vi "Front Panel Tyler SYNCHRONIZED.vi"() -> ()   [LabVIEW 2017, in "LD Reading.lvclass"]
uses:
  LD Reading.lvclass
  Experimental Parameters.ctl
  Reference Channel Intensities.ctl
  Sample Channel Intensities.ctl
  Realtime Output.ctl
  Average Data.ctl
  LD Reading.lvclass/LD Reading.ctl
  MCTypedef.ctl
  <vilib>/Instr/_visa.llb/VISA Configure Serial Port (Instr).vi
  <vilib>/Utility/file.llb/Write Delimited Spreadsheet (string).vi
  <vilib>/Utility/inputDevices.llb/keyboardAcquire.vi
panel:
  in  "Experimental Controls":enum32{"Page 1", "Page 2"}(tab)
  in  "Collect Data":bool
  out "Running":bool
  in  "Save Measurements?":bool
  in  "Stop and Discard \nMeasurement":bool
  in  "Output Filename (stem)":path
  out "Finished":bool
  in  "Selected Reference Channel":enum32{"Channel 1", "Channel 2", "Channel 3"}(radio)
  in  "Selected Sample Channel":enum32{"Channel 1", "Channel 2", "Channel 3"}(radio)
  in  "Data Collection Mode":enum32{"Reference", "Sample"}(radio)
  in  "Export Data":bool
  in  "Enable Translation Stage":bool
  in  "Shutter Control":bool
  out "error out":errorcluster
  in  "clear":bool
  in  "sp33d":dbl(knob)=0.5 step=0.5 scale=0.5..1.0
  out "read buffer":string
  out "Data Collection Progress":u8(slide) scale=0.0..100.0
  out "Current Phase":string
  in  "?":T1(tab)
  out "Diode/PMT":cluster{dbl[], dbl[]}(graph)
  out "RMS Voltage":cluster{dbl[], dbl[]}(graph)
  out "Photodiode Voltage  (V)":cluster{dbl[], dbl[]}(graph)
  out "PMT Voltage":cluster{dbl[], dbl[]}(graph)
  out "Reference Averages":T2
  out "Sample Averages":T2
  out "Realtime Output":T3
  out "Sample Analysis":T4
  out "Reference Analysis":T5
  in  "Experimental Parameters":T6={"Correction Factor"=2.9405, "Data Interval (s)"=1.0, "Number of Data Points"=60.0, "Incident Angle (Degrees)"=63.0, "Refractive Index (Rare)"=1.335, "Refractive Index (Dense)"=1.55222, "PMT Bias Voltage (V)"=0.0, "Laser Wavelength (nm)"=0.0, "Preamplifier Output Gain (uA/V)"=10.0, "PEM Monitoring Frequency"=2} {"PEM Monitoring Frequency" min=1 max=2 step=1}
  in  "stop":bool
  # "Dichroism Controller"
  # "Data Collection Parameters"
  # "System Settings"
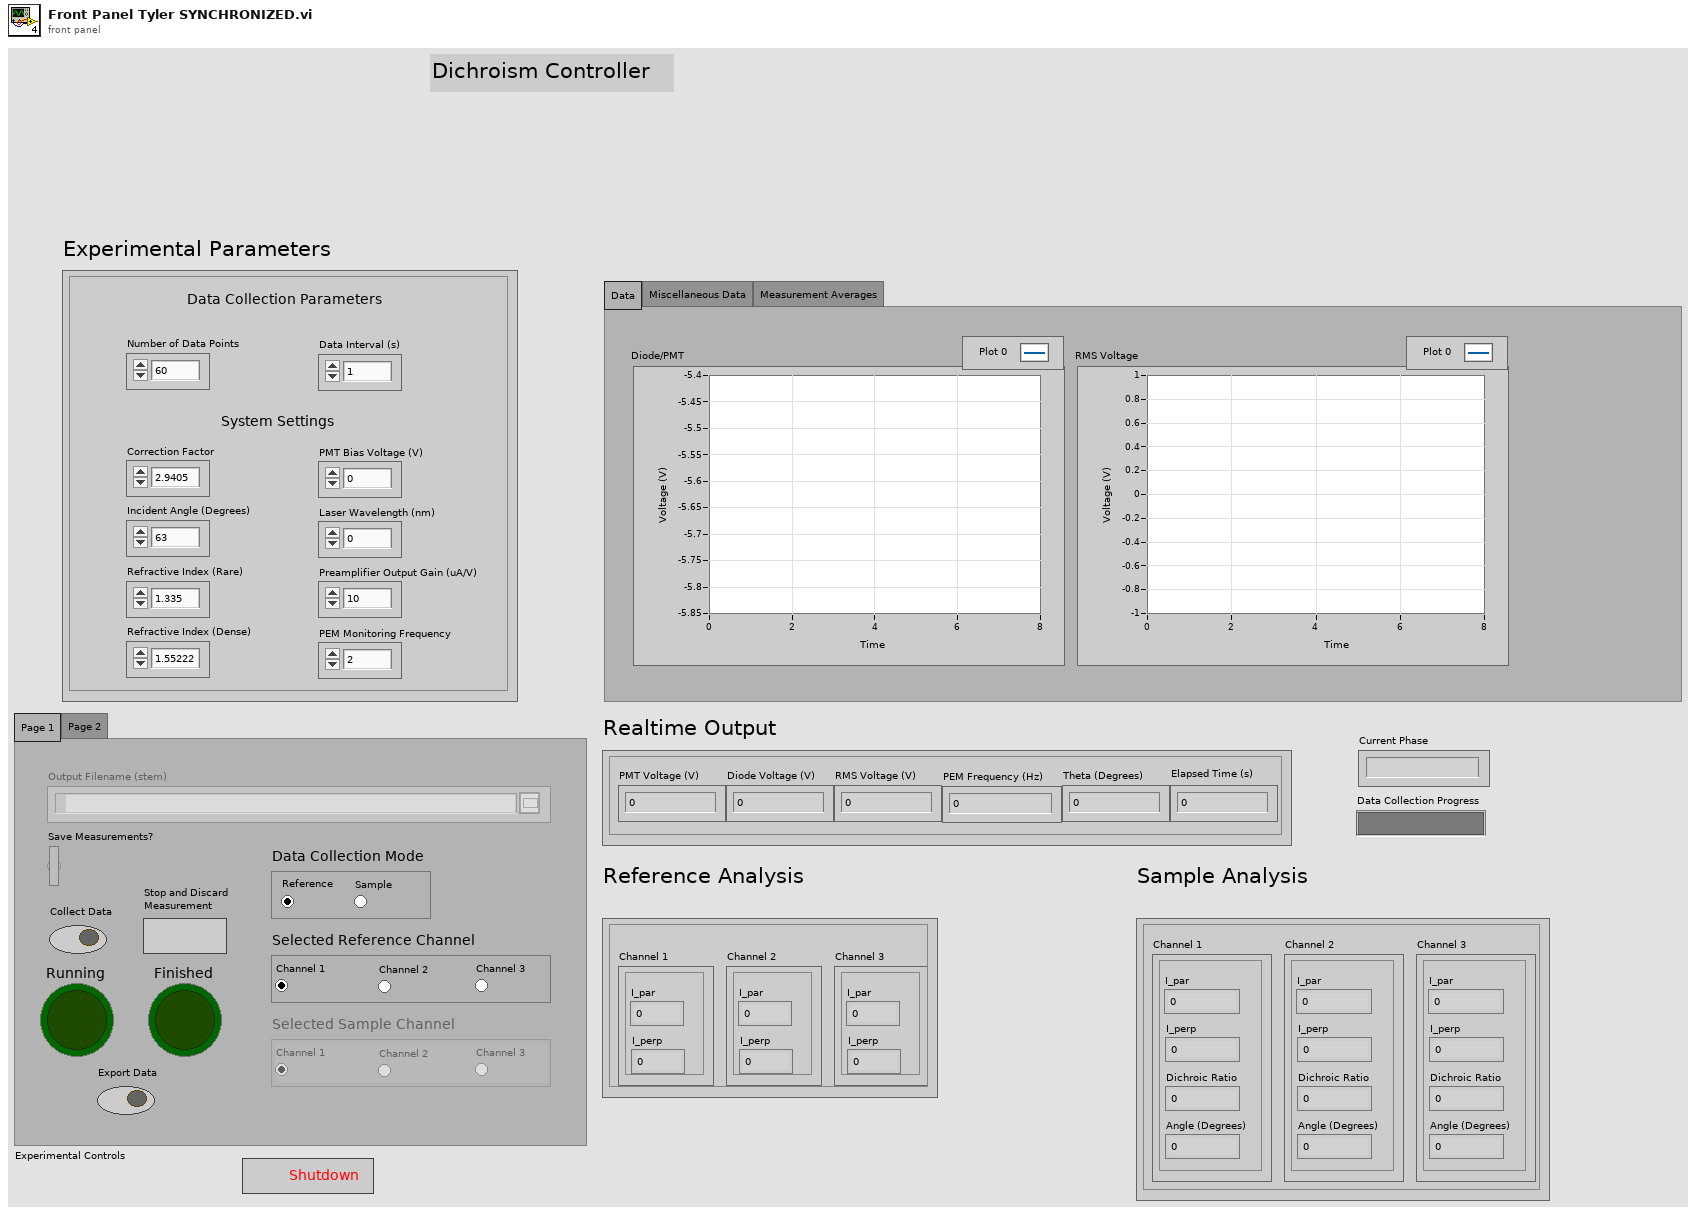
[diagram p1: front panel]
types:
  T1 = enum32{"Data", "Miscellaneous Data", "Measurement Averages"}
  T2 = typedef "Average Data.ctl" = cluster{"Channel 1":cluster{"PMT Voltage (V)":dbl, "Photodiode Voltage (V)":dbl, "RMS Voltage (V)":dbl, "Theta (Degrees)":dbl}, "Channel 2":cluster{"PMT Voltage (V)":dbl, "Photodiode Voltage (V)":dbl, "RMS Voltage (V)":dbl, "Theta (Degrees)":dbl}, "Channel 3":cluster{"PMT Voltage (V)":dbl, "Photodiode Voltage (V)":dbl, "RMS Voltage (V)":dbl, "Theta (Degrees)":dbl}}
  T3 = typedef "Realtime Output.ctl" = cluster{"Elapsed Time (s)":dbl, "PMT Voltage (V)":dbl, "Diode Voltage (V)":dbl, "RMS Voltage (V)":dbl, "Theta (Degrees)":dbl, "PEM Frequency (Hz)":dbl}
  T4 = typedef "Sample Channel Intensities.ctl" = cluster{"Channel 1":cluster{"I_par":dbl, "I_perp":dbl, "Dichroic Ratio":dbl, "Angle (Degrees)":dbl}, "Channel 2":cluster{"I_par":dbl, "I_perp":dbl, "Dichroic Ratio":dbl, "Angle (Degrees)":dbl}, "Channel 3":cluster{"I_par":dbl, "I_perp":dbl, "Dichroic Ratio":dbl, "Angle (Degrees)":dbl}}
  T5 = typedef "Reference Channel Intensities.ctl" = cluster{"Channel 1":cluster{"I_par":dbl, "I_perp":dbl}, "Channel 2":cluster{"I_par":dbl, "I_perp":dbl}, "Channel 3":cluster{"I_par":dbl, "I_perp":dbl}}
  T6 = typedef "Experimental Parameters.ctl" = cluster{"Correction Factor":dbl, "Data Interval (s)":dbl, "Number of Data Points":dbl, "Incident Angle (Degrees)":dbl, "Refractive Index (Rare)":dbl, "Refractive Index (Dense)":dbl, "PMT Bias Voltage (V)":dbl, "Laser Wavelength (nm)":dbl, "Preamplifier Output Gain (uA/V)":dbl, "PEM Monitoring Frequency":u8}
  T7 = enum8{"Enabled", "Disabled", "Disabled and Grayed Out"}
  T8 = typedef "MCTypedef.ctl" = enum16{"idle", "forward", "reverse", "clear"}
  T9 = cluster{dbl[], dbl[], dbl[], dbl[], dbl[], dbl[], dbl[]}
  T10 = cluster{"RMS Voltage Array":dbl[], "Photodiode Voltage Array":dbl[], "PMT Voltage Array":dbl[], "Diode/PMT Ratio Array":dbl[], "Time Array":dbl[], "PEM Frequency Array":dbl[], "Theta Array":dbl[]}
  T11 = cluster{"PMT Voltage (V)":dbl, "Photodiode Voltage (V)":dbl, "RMS Voltage (V)":dbl, "Theta (Degrees)":dbl}
  T12 = cluster{"I_par":dbl, "I_perp":dbl, "Dichroic Ratio":dbl, "Angle (Degrees)":dbl}
  T13 = typedef "NI_Matrix.lvlib/RealMatrix.ctl" = dbl[][]
  T14 = enum16{"0", "1", "2", "3", "4", "5", "6", "7", "8", "9", "A", "B", "C", "D", "E", "F", "G", "H", "I", "J", "K", "L", "M", "N", "O", "P", "Q", "R", "S", "T", "U", "V", "W", "X", "Y", "Z", "F1", "F2", "F3", "F4", "F5", "F6", "F7", "F8", "F9", "F10", "F11", "F12", "F13", "F14", "F15", "ADD", "BACK", "BACKSLASH", "CAPITAL", "COMMA", "DECIMAL", "DELETE", "DIVIDE", "DOWN", "END", "EQUALS", "ESCAPE", "GRAVE (`)", "HOME", "INSERT", "LBRACKET", "LCONTROL", "LEFT", "L ALT", "LSHIFT", "LWIN", "MINUS", "MULTIPLY", "NEXT", "NUMLOCK", "NUMPAD_0", "NUMPAD_1", "NUMPAD_2", "NUMPAD_3", "NUMPAD_4", "NUMPAD_5", "NUMPAD_6", "NUMPAD_7", "NUMPAD_8", "NUMPAD_9", "PAUSE", "PERIOD", "PRIOR (PG UP)", "RBRACKET", "RCONTROL", "RETURN", "RIGHT", "R ALT", "RSHIFT", "RWIN", "SCROLL", "SEMICOLON", "SLASH", "SPACE", "SUBTRACT", "TAB", "UP", "ENTER (num pad)", "' (quote)"}[]
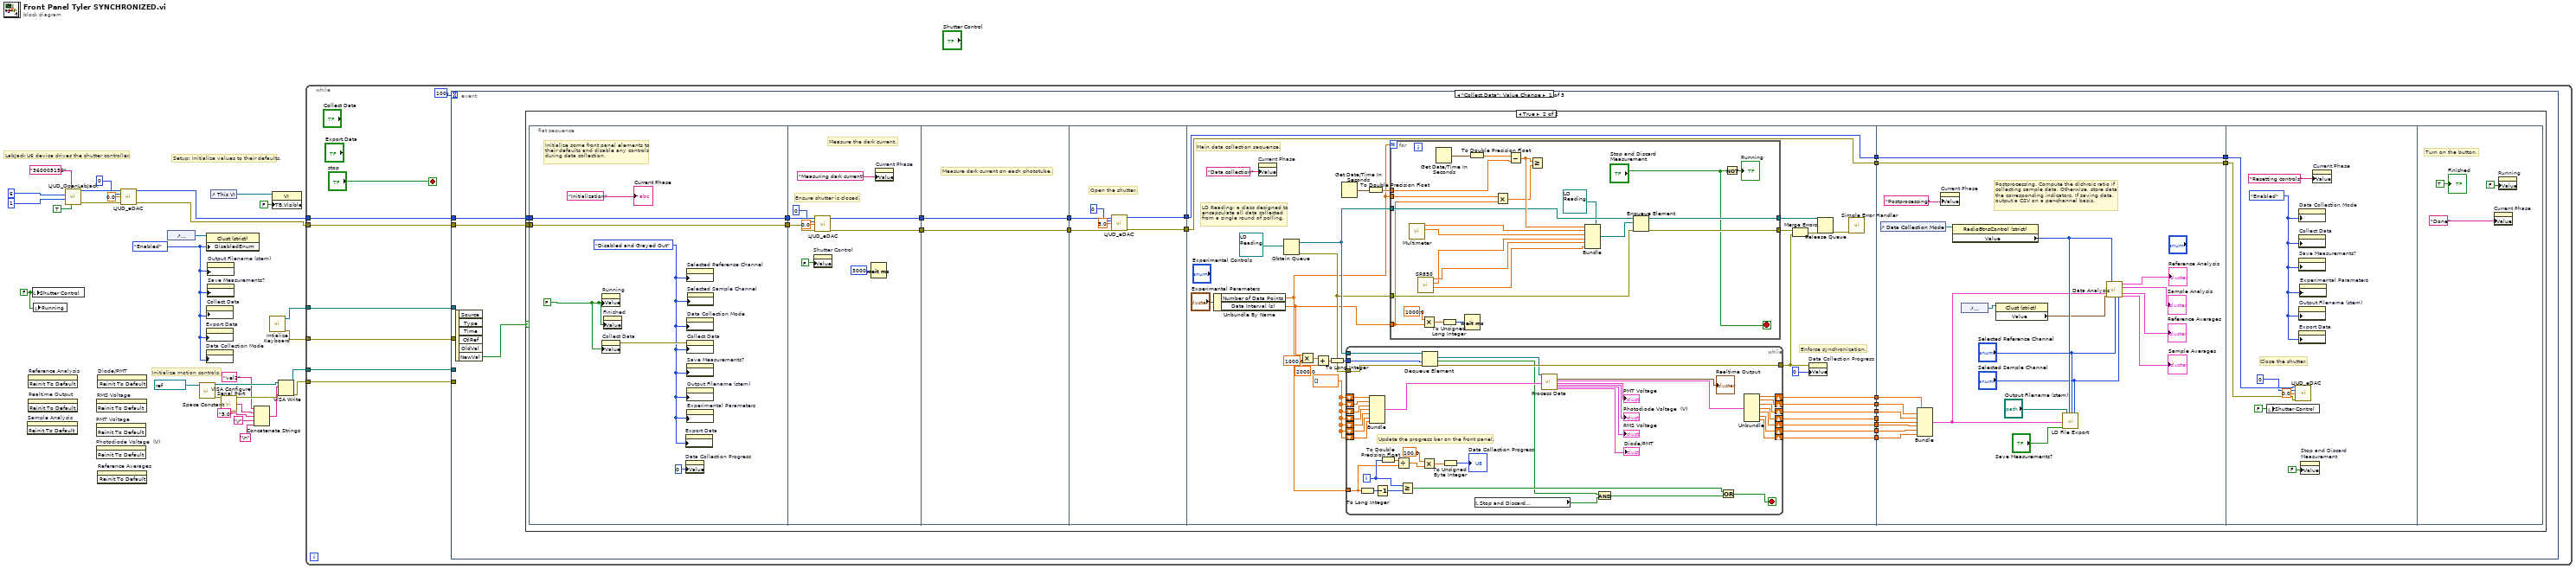
[diagram p0: block diagram]
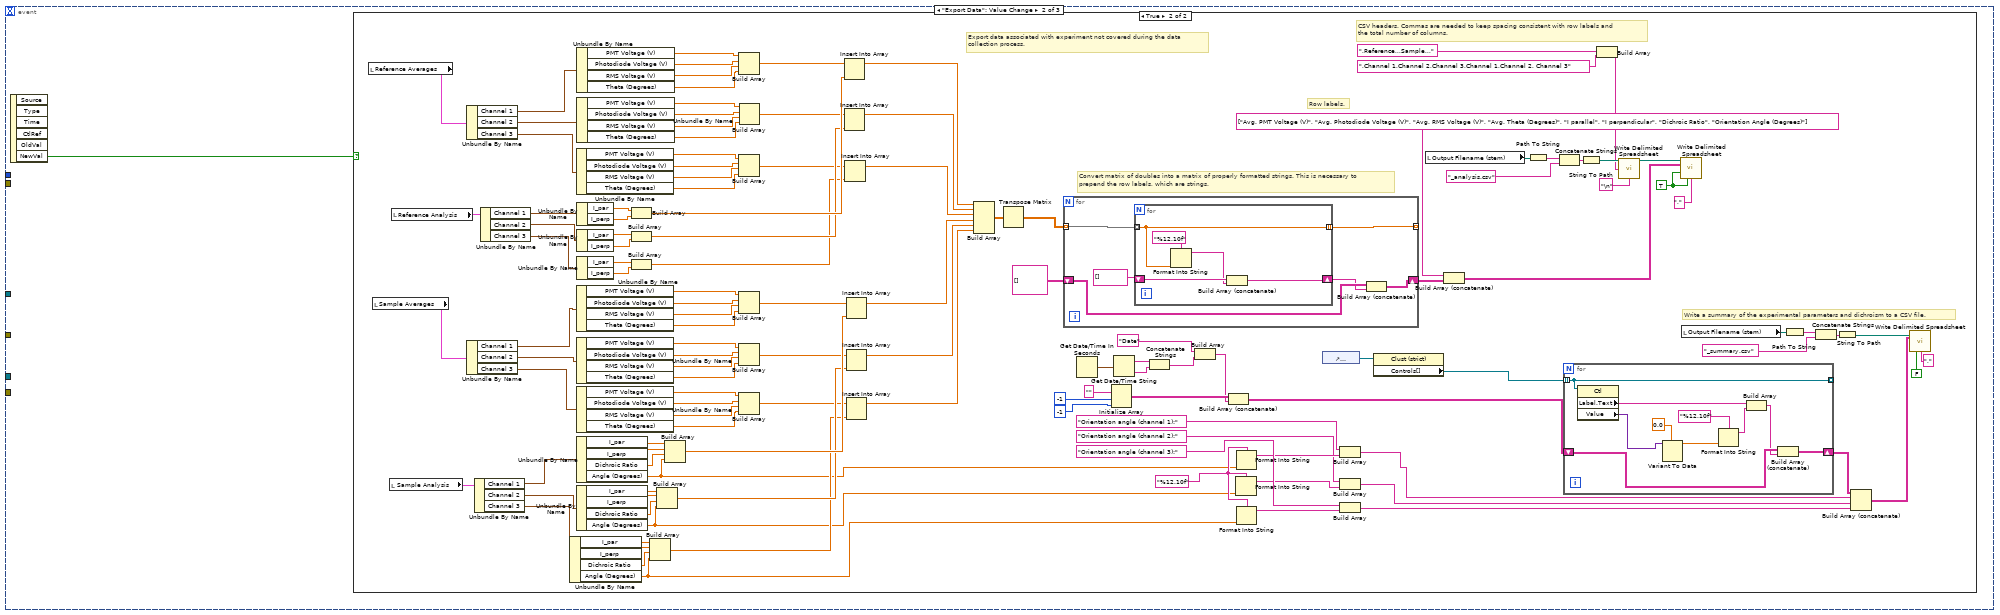
[diagram p3: hidden frame]
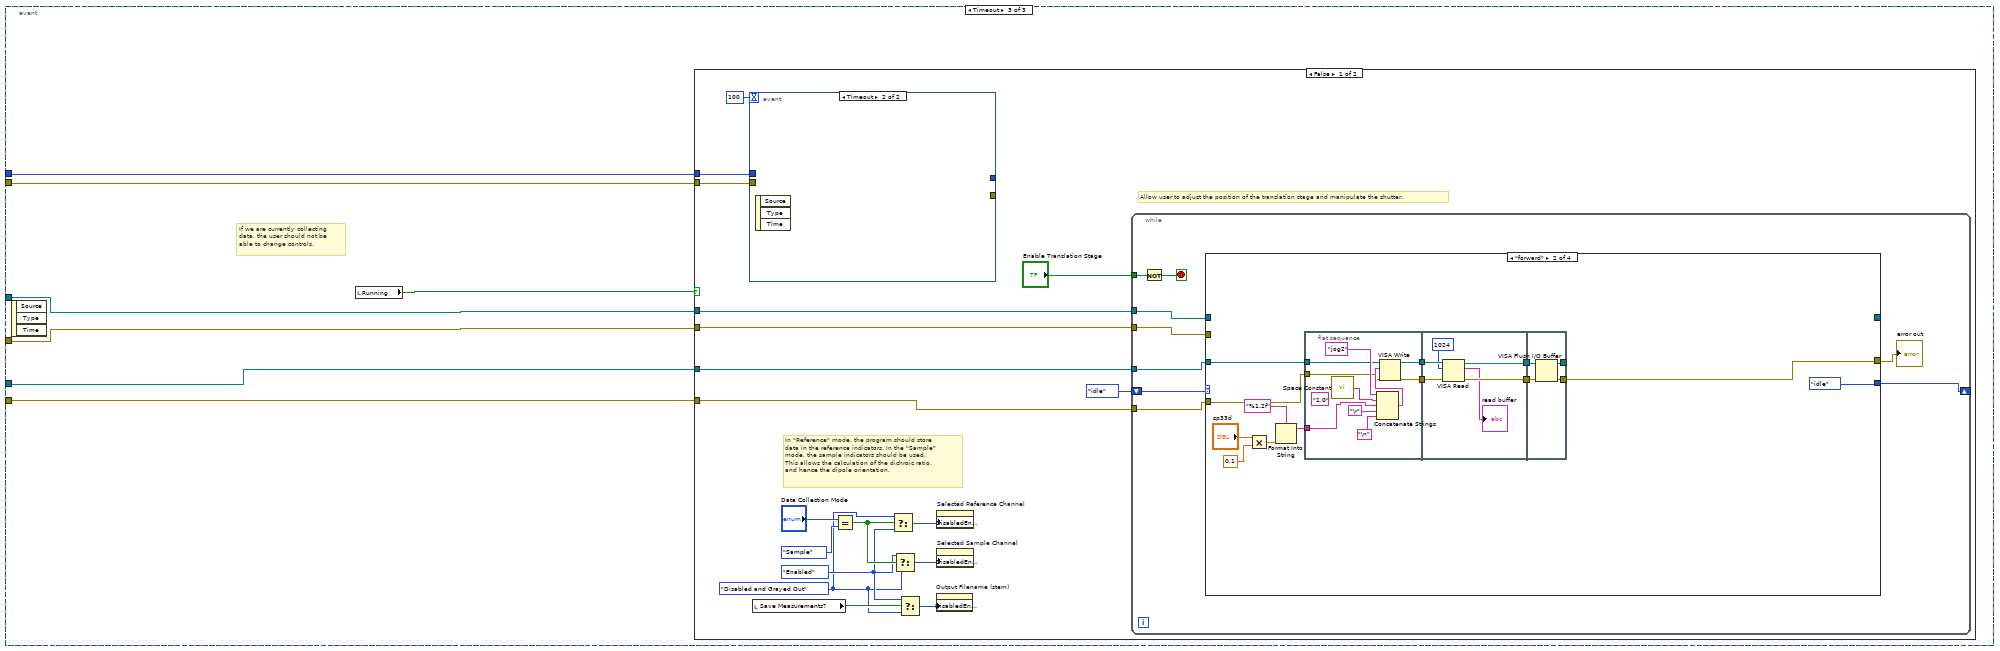
[diagram p5: hidden frame]
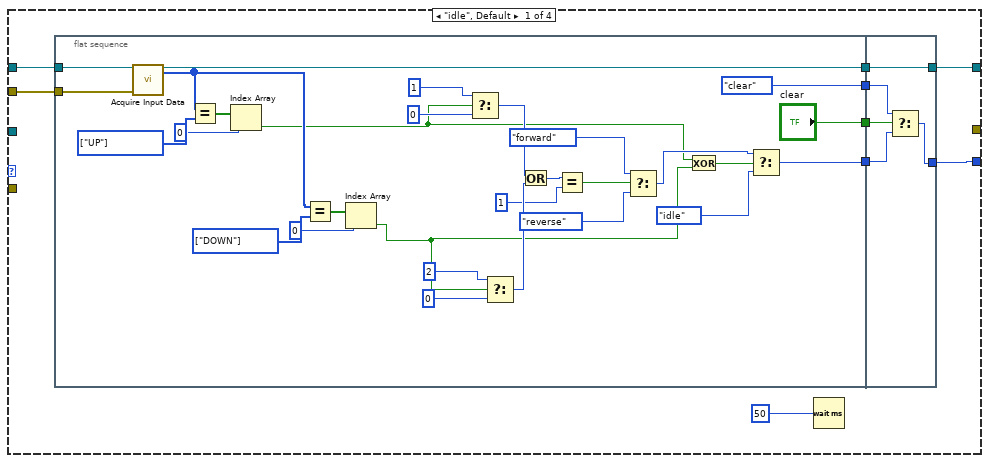
[diagram p6: hidden frame]
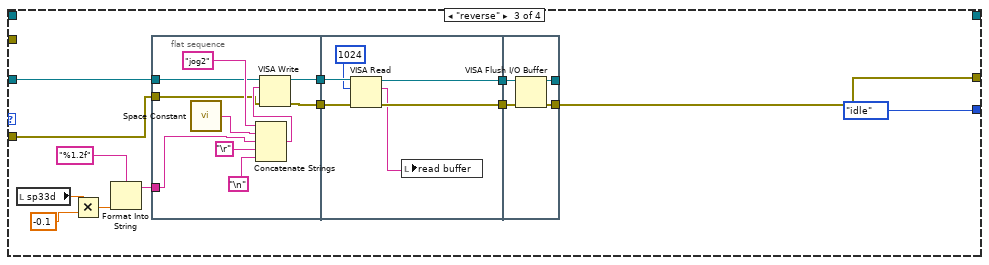
[diagram p7: hidden frame]
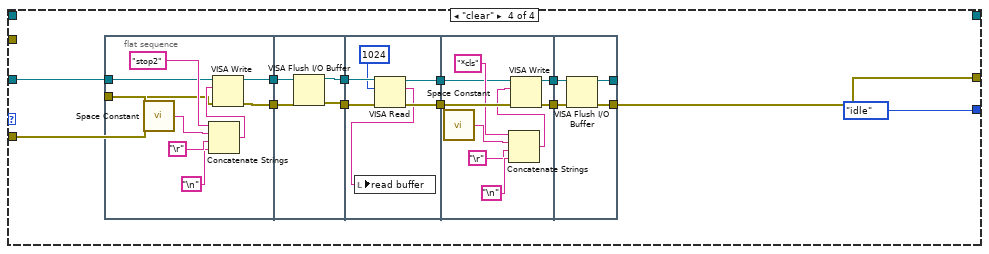
[diagram p8: hidden frame]
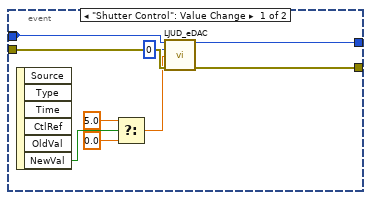
[diagram p9: hidden frame]
diagram:
  w1 = FALSE ("Shutter Control")
  w25 = T7."Enabled" ("Disabled")
  # "LabJack U6 device drives the shutter controller."
  # "Initialize motion controls."
  # "Setup: Initialize values to their defaults."
  n1 = invoke on="Sample Analysis" class="Clust (strict)" method="Reinit To Default"() -> ()  [unwired: 3 in, 3 out]
  n2 = invoke on="Reference Analysis" class="Clust (strict)" method="Reinit To Default"() -> ()  [unwired: 3 in, 3 out]
  n3 = invoke on="Realtime Output" class="Clust (strict)" method="Reinit To Default"() -> ()  [unwired: 3 in, 3 out]
  n4 = local write "Shutter Control"(w1) -> ()
  n5 = local write "Running"(w1) -> ()
  n6 = call "LJUD_OpenLabJack.vi"("FirstFound"=TRUE, "Address"="360005150", "ConnectionType"=1, "DeviceType"=6) -> ("error out"=w6:errorcluster, "Handle"=w7:i32)  [unwired: 6 in]
  n7 = invoke on="PMT Voltage" class="XYGraph (strict)" method="Reinit To Default"() -> ()  [unwired: 3 in, 3 out]
  n8 = invoke on="Photodiode Voltage  (V)" class="XYGraph (strict)" method="Reinit To Default"() -> ()  [unwired: 3 in, 3 out]
  n9 = invoke on="RMS Voltage" class="XYGraph (strict)" method="Reinit To Default"() -> ()  [unwired: 3 in, 3 out]
  n10 = invoke on="Diode/PMT" class="XYGraph (strict)" method="Reinit To Default"() -> ()  [unwired: 3 in, 3 out]
  n11 = invoke on="Reference Averages" class="Clust (strict)" method="Reinit To Default"() -> ()  [unwired: 3 in, 3 out]
  n12 = call "LJUD_eDAC.vi"("Handle In"=w7, "Channel"=0, "Voltage"=0.0, "error in"=w6) -> ("Handle Out"=w5:i32, "error out"=w4:errorcluster)  [unwired: 10 in]
  n13 = control-ref of="Experimental Parameters"() -> (w26:refnum<vi>)
  n14 = call-poly "VISA Configure Serial Port"("VISA resource name"=refnum<visa-resource-name> "COM1") -> ("VISA resource name out"=w23:refnum<visa-resource-name>, "error out"=w24:errorcluster)  [unwired: 13 in]
  n15 = property on="Export Data" class="Bool"("DisabledEnum"=w25) -> ()  [unwired: 2 in, 2 out]
  n16 = property on="Data Collection Mode" class="RadioBtnsControl (strict)"("DisabledEnum"=w25) -> ()  [unwired: 2 in, 2 out]
  n17 = property class="Clust (strict)"(reference=w26, "DisabledEnum"=w25) -> ()  [unwired: 1 in, 2 out]
  n18 = property on="Collect Data" class="Bool (strict)"("DisabledEnum"=w25) -> ()  [unwired: 2 in, 2 out]
  n19 = property on="Output Filename (stem)" class="Path"("DisabledEnum"=w25) -> ()  [unwired: 2 in, 2 out]
  n20 = property on="Save Measurements?" class="Bool (strict)"("DisabledEnum"=w25) -> ()  [unwired: 2 in, 2 out]
  n21 = control-ref of="This VI"() -> (w27:refnum<vi>)
  n22 = call <vilib>:"Space Constant.vi"() -> ("String"=w22:string)
  n23 = Concatenate Strings("vel2" ("string"), w22, "5.0" ("string"), "\r", "\n") -> (w21:string)
  n24 = call <vilib>:"Intialize Keyboard.vi"() -> ("error out"=w13:errorcluster, "device ID"=w12:refnum<k1>)  [unwired: 10 in]
  n25 = property class="VI"(reference=w27, "TB.Visible"=FALSE ("Tool Bar:Visible")) -> ()  [unwired: 1 in, 2 out]
  n26 = VISA Write(VISA resource name=w23, write buffer=w21, error in (no error)=w24) -> (VISA resource name out=w14:refnum<visa-resource-name>, error out=w15:errorcluster)  [unwired: 1 out]
  n27 = while {
    tunnel: w15 -> [w34]
    tunnel: w14 -> [w33]
    tunnel: w13 -> [w32]
    tunnel: w12 -> [w31]
    tunnel: w5 -> [w30]
    tunnel: w4 -> [w29]
    stop <- "stop" stop-if-true
    n28 = event shown="[0] \"Collect Data\": Value Change" {
      selector: _ -> [_ _ _]
      dyn-events: _ -> [_ _ _]
      timeout: 100 -> [_ _ _]
      tunnel: w34 -> [_ _ w365]
      tunnel: w33 -> [_ _ w364]
      tunnel: w32 -> [_ _ w363]
      tunnel: w31 -> [_ _ w362]
      tunnel: w30 -> [w38 _ w361]
      tunnel: w29 -> [w37 _ w360]
      event "Collect Data": Value Change {
        n29 = event-data() -> ("NewVal"=w39:bool)  [unwired: 1 in, 5 out]
        n30 = case shown="True" w39 {
          tunnel: w38 -> [_ w52]
          tunnel: w37 -> [_ w50]
          frame False {
          }
          frame True {
            n31 = flat-sequence {
              tunnel: [w62] -> w53
              tunnel: w52 -> [w62]
              tunnel: [w61] -> w51
              tunnel: w50 -> [w61]
              tunnel: w53 -> [w76]
              tunnel: w51 -> [w75]
              tunnel: [w71] -> w49
              tunnel: [w70] -> w48
              tunnel: w49 -> [w78]
              tunnel: w48 -> [w77]
              tunnel: [w78] -> w47
              tunnel: [w77] -> w46
              tunnel: w47 -> [w84]
              tunnel: w46 -> [w83]
              tunnel: [w80] -> w45
              tunnel: [w79] -> w44
              tunnel: [w104] -> w60
              tunnel: [w103] -> w59
              tunnel: [w102] -> w58
              tunnel: [w105] -> w57
              tunnel: [w101] -> w56
              tunnel: [w100] -> w55
              tunnel: [w95] -> w54
              tunnel: w45 -> [w86]
              tunnel: w44 -> [w85]
              tunnel: [w86] -> w42
              tunnel: [w85] -> w41
              tunnel: w60 -> [w196]
              tunnel: w59 -> [w195]
              tunnel: w58 -> [w194]
              tunnel: w57 -> [w197]
              tunnel: w56 -> [w193]
              tunnel: w55 -> [w192]
              tunnel: w54 -> [w191]
              tunnel: [w179] -> w43
              tunnel: w42 -> [w179]
              tunnel: w41 -> [w178]
              tunnel: [w178] -> w40
              tunnel: w43 -> [w204]
              tunnel: w40 -> [w203]
              frame #0 {
                w63 = T7."Disabled and Grayed Out" ("Disabled")
                w64 = FALSE
                # "Initialize some front panel elements to \ntheir defaults and disable any controls \nduring data collection."
                n32 = property on="Running" class="Bool (strict)"("Value"=w64) -> ()  [unwired: 2 in, 2 out]
                n33 = property on="Collect Data" class="Bool (strict)"("Value"=w64) -> (error out=w67:errorcluster)  [unwired: 2 in, 1 out]
                n34 = property on="Finished" class="Bool (strict)"("Value"=w64) -> ()  [unwired: 2 in, 2 out]
                n35 = property on="Export Data" class="Bool"("DisabledEnum"=w63) -> ()  [unwired: 2 in, 2 out]
                n36 = property on="Data Collection Progress" class="Slide (strict)"("Value"=u8 0 ("Progress")) -> ()  [unwired: 2 in, 2 out]
                n37 = property on="Selected Reference Channel" class="RadioBtnsControl (strict)"("DisabledEnum"=w63) -> ()  [unwired: 2 in, 2 out]
                n38 = property on="Data Collection Mode" class="RadioBtnsControl (strict)"("DisabledEnum"=w63) -> ()  [unwired: 2 in, 2 out]
                n39 = property on="Collect Data" class="Bool (strict)"(error in=w67, "DisabledEnum"=w63) -> ()  [unwired: 1 in, 2 out]
                n40 = property on="Save Measurements?" class="Bool (strict)"("DisabledEnum"=w63) -> ()  [unwired: 2 in, 2 out]
                n41 = property on="Output Filename (stem)" class="Path"("DisabledEnum"=w63) -> ()  [unwired: 2 in, 2 out]
                n42 = property on="Experimental Parameters" class="Clust (strict)"("DisabledEnum"=w63) -> ()  [unwired: 2 in, 2 out]
                n43 = property on="Selected Sample Channel" class="RadioBtnsControl (strict)"("DisabledEnum"=w63) -> ()  [unwired: 2 in, 2 out]
                "Current Phase" <- "Initialization"
              }
              frame #1 {
                # "Ensure shutter is closed."
                # "Measure the dark current."
                n44 = property on="Shutter Control" class="Bool (strict)"("Value"=FALSE ("Shutter Control")) -> ()  [unwired: 2 in, 2 out]
                n45 = call "LJUD_eDAC.vi"("Handle In"=w76, "Channel"=0, "Voltage"=0.0, "error in"=w75) -> ("Handle Out"=w71:i32, "error out"=w70:errorcluster)  [unwired: 10 in]
                n46 = Wait (ms)(milliseconds to wait=u32 3000) -> ()  [unwired: 1 out]
                n47 = property on="Current Phase" class="Str"("Value"="Measuring dark current") -> ()  [unwired: 2 in, 2 out]
              }
              frame #2 {
                # "Measure dark current on each phototube."
              }
              frame #3 {
                # "Open the shutter."
                n48 = call "LJUD_eDAC.vi"("Handle In"=w84, "Channel"=0, "Voltage"=5.0, "error in"=w83) -> ("Handle Out"=w80:i32, "error out"=w79:errorcluster)  [unwired: 10 in]
              }
              frame #4 {
                w96 = dbl[] []
                # "Enforce synchronization."
                # "Main data collection sequence."
                # "LD Reading: a class designed to \nencapsulate all data collected \nfrom a single round of polling."
                n49 = Unbundle By Name("Experimental Parameters") -> ("Number of Data Points"=w93:dbl, "Data Interval (s)"=w92:dbl)
                n50 = property on="Current Phase" class="Str"("Value"="Data collection") -> ()  [unwired: 2 in, 2 out]
                n51 = Obtain Queue(element data type=refnum<class "LD Reading.lvclass"> refnum ("LD Reading.lvclass")) -> (queue out=w111:refnum<queue>, error out=w110:errorcluster)  [unwired: 4 in, 1 out]
                n52 = Multiply(x=w92, y=1000.0) -> (x*y=w90:dbl)
                n53 = Add(x=w90, y=2000.0) -> (x+y=w88:dbl)
                n54 = To Long Integer(number=w88) -> (32bit integer=w87:i32)
                n55 = Get Date/Time In Seconds() -> (seconds since 1Jan1904=w114:timestamp)
                n56 = while {
                  tunnel: w111 -> [w177]
                  shift-right: [w156] -> w105
                  shift-left: w96 -> [w163]
                  shift-right: [w155] -> w104
                  shift-left: w96 -> [w162]
                  shift-right: [w154] -> w103
                  shift-left: w96 -> [w161]
                  shift-right: [w153] -> w102
                  shift-left: w96 -> [w160]
                  shift-right: [w152] -> w101
                  shift-left: w96 -> [w159]
                  shift-right: [w151] -> w100
                  shift-left: w96 -> [w158]
                  shift-right: [w150] -> w95
                  shift-left: w96 -> [w157]
                  tunnel: w110 -> [w175]
                  tunnel: [w174] -> w98
                  tunnel: w93 -> [w164]
                  tunnel: w87 -> [w138]
                  i -> [w169]
                  stop <- w176 stop-if-true
                  # "Update the progress bar on the front panel."
                  n57 = To Long Integer(number=w164) -> (32bit integer=w170:i32)
                  n58 = Bundle(w163, w162, w161, w160, w159, w158, w157) -> (w148:T9)  [unwired: 1 in]
                  n59 = Decrement(x=w170) -> (x-1=w173:i32)
                  n60 = To Double Precision Float(number=w169) -> (double precision float=w168:dbl)
                  n61 = Divide(x=w168, y=w164) -> (x/y=w171:dbl)
                  n62 = Greater Or Equal?(x=w169, y=w173) -> (x >= y?=w172:bool)
                  n63 = Multiply(x=100.0, y=w171) -> (x*y=w166:dbl)
                  n64 = Dequeue Element(queue=w177, timeout in ms (-1)=w138, error in (no error)=w175) -> (element=w149:refnum<class "LD Reading.lvclass">, timed out?=w141:bool, error out=w174:errorcluster)  [unwired: 1 out]
                  n65 = To Unsigned Byte Integer(number=w166) -> (unsigned 8bit integer=→"Data Collection Progress":u8)
                  n66 = local read "Stop and Discard \nMeasurement"() -> (w140:bool)
                  n67 = call "Process Data.vi"("LD Reading in"=w149, "Input Cluster"=w148) -> ("Realtime Output"=→"Realtime Output":T3, "Output Cluster"=w146:T10, "PMT Voltage (V)"=→"PMT Voltage":cluster{dbl[], dbl[]}, "Photodiode Voltage  (V)"=→"Photodiode Voltage  (V)":cluster{dbl[], dbl[]}, "RMS Voltage (mV)"=→"RMS Voltage":cluster{dbl[], dbl[]}, "Diode/PMT"=→"Diode/PMT":cluster{dbl[], dbl[]})  [unwired: 20 in]
                  n68 = And(x=w141, y=w140) -> (x .and. y?=w139:bool)
                  n69 = Or(x=w172, y=w139) -> (x .or. y?=w176:bool)
                  n70 = Unbundle(w146) -> ("RMS Voltage Array"=w156:dbl[], "Photodiode Voltage Array"=w155:dbl[], "PMT Voltage Array"=w154:dbl[], "Diode/PMT Ratio Array"=w153:dbl[], "Time Array"=w152:dbl[], "PEM Frequency Array"=w151:dbl[], "Theta Array"=w150:dbl[])
                }
                n71 = To Double Precision Float(number=w114) -> (double precision float=w113:dbl)
                n72 = for {
                  N: w93 -> [_]
                  tunnel: w92 -> [w118]
                  tunnel: w113 -> [w127]
                  tunnel: w111 -> [w134]
                  tunnel: [w131] -> w106
                  tunnel: w110 -> [w129]
                  tunnel: [w128] -> w109
                  tunnel: w93 -> [w126]
                  stop <- "Stop and Discard \nMeasurement" stop-if-true
                  n73 = call "Multimeter.vi"() -> ("Voltage 2"=w115:dbl, "Voltage"=w121:dbl)  [unwired: 9 in, 1 out]
                  n74 = call "SR850.vi"() -> ("Frequency"=w122:dbl, "R"=w123:dbl, "Theta"=w124:dbl)  [unwired: 8 in, 1 out]
                  n75 = Multiply(x=1000.0, y=w118) -> (x*y=w120:dbl)
                  n76 = Get Date/Time In Seconds() -> (seconds since 1Jan1904=w137:timestamp)
                  n77 = To Unsigned Long Integer(number=w120) -> (unsigned 32bit integer=w117:u32)
                  n78 = Wait (ms)(milliseconds to wait=w117) -> ()  [unwired: 1 out]
                  n79 = To Double Precision Float(number=w137) -> (double precision float=w136:dbl)
                  n80 = Multiply(x=w126, y=w118) -> (x*y=w125:dbl)
                  n81 = Subtract(x=w136, y=w127) -> (x-y=w135:dbl)
                  n82 = Greater Or Equal?(x=w135, y=w125) -> ()  [unwired: 1 out]
                  n83 = Bundle(cluster=refnum<class "LD Reading.lvclass"> refnum ("LD Reading.lvclass"), w135, w121, w115, w123, w124, w122) -> (w132:refnum<class "LD Reading.lvclass">)
                  n84 = Enqueue Element(queue=w134, element=w132, error in (no error)=w129) -> (queue out=w131:refnum<queue>, error out=w128:errorcluster)  [unwired: 1 in, 1 out]
                  n85 = Not(x="Stop and Discard \nMeasurement") -> (.not. x?=→"Running":bool)
                }
                n86 = Merge Errors(w109, w98) -> (w108:errorcluster)
                n87 = property on="Data Collection Progress" class="Slide (strict)"(error in=w98, "Value"=u8 0 ("Progress")) -> ()  [unwired: 1 in, 2 out]
                n88 = Release Queue(queue=w106, error in (no error)=w108) -> (error out=w107:errorcluster)  [unwired: 1 in, 2 out]
                n89 = call <vilib>:"Simple Error Handler.vi"("error in (no error)"=w107) -> ()  [unwired: 4 in, 5 out]
              }
              frame #5 {
                # "Postprocessing. Compute the dichroic ratio if \ncollecting sample data. Otherwise, store data \nthe corresponding indicators. If saving data, \noutput a CSV on a per-channel basis."
                n90 = control-ref of="Data Collection Mode"() -> (w190:refnum<vi>)
                n91 = Bundle(w197, w196, w195, w194, w193, w192, w191) -> (w182:T9)  [unwired: 1 in]
                n92 = property on="Current Phase" class="Str"("Value"="Postprocessing") -> ()  [unwired: 2 in, 2 out]
                n93 = property class="RadioBtnsControl (strict)"(reference=w190) -> ("Value"=w185:enum32{"Reference", "Sample"})  [unwired: 1 in, 2 out]
                n94 = control-ref of="Experimental Parameters"() -> (w181:refnum<vi>)
                n95 = property class="Clust (strict)"(reference=w181) -> ("Value"=w180:T6)  [unwired: 1 in, 2 out]
                n96 = call "LD File Export.vi"("Input Cluster"=w182, "Save Data?"="Save Measurements?", "Output Filename (stem)"="Output Filename (stem)", "Data Collection Mode"=w185, "Selected Reference Channel"="Selected Reference Channel", "Selected Sample Channel"="Selected Sample Channel") -> ()  [unwired: 14 in]
                n97 = call "Data Analysis.vi"("Data Collection Mode"=w185, "Cluster"=w182, "Experimental Parameters"=w180, "Selected Reference Channel in"="Selected Reference Channel", "Selected Sample Channel in"="Selected Sample Channel") -> ("Reference Analysis"=→"Reference Analysis":T5, "Sample Analysis"=→"Sample Analysis":T4, "Reference Averages"=→"Reference Averages":T2, "Sample Averages"=→"Sample Averages":T2)  [unwired: 7 in]
              }
              frame #6 {
                w206 = T7."Enabled" ("Disabled")
                # "Close the shutter."
                n98 = local write "Shutter Control"(FALSE ("Shutter Control")) -> ()
                n99 = call "LJUD_eDAC.vi"("Handle In"=w204, "Channel"=0, "Voltage"=0.0, "error in"=w203) -> ()  [unwired: 10 in, 2 out]
                n100 = property on="Data Collection Mode" class="RadioBtnsControl (strict)"("DisabledEnum"=w206) -> ()  [unwired: 2 in, 2 out]
                n101 = property on="Collect Data" class="Bool (strict)"("DisabledEnum"=w206) -> ()  [unwired: 2 in, 2 out]
                n102 = property on="Save Measurements?" class="Bool (strict)"("DisabledEnum"=w206) -> ()  [unwired: 2 in, 2 out]
                n103 = property on="Output Filename (stem)" class="Path"("DisabledEnum"=w206) -> ()  [unwired: 2 in, 2 out]
                n104 = property on="Export Data" class="Bool"("DisabledEnum"=w206) -> ()  [unwired: 2 in, 2 out]
                n105 = property on="Experimental Parameters" class="Clust (strict)"("DisabledEnum"=w206) -> ()  [unwired: 2 in, 2 out]
                n106 = property on="Stop and Discard \nMeasurement" class="Bool (strict)"("Value"=FALSE ("Stop Data Collection")) -> ()  [unwired: 2 in, 2 out]
                n107 = property on="Current Phase" class="Str"("Value"="Resetting controls") -> ()  [unwired: 2 in, 2 out]
              }
              frame #7 {
                # "Turn on the button."
                n108 = property on="Current Phase" class="Str"("Value"="Done") -> ()  [unwired: 2 in, 2 out]
                n109 = property on="Running" class="Bool (strict)"("Value"=FALSE ("Running")) -> ()  [unwired: 2 in, 2 out]
                "Finished" <- TRUE ("Finished")
              }
            }
          }
        }
      }
      event "Export Data": Value Change {
        n110 = event-data() -> ("NewVal"=w212:bool)  [unwired: 1 in, 5 out]
        n111 = case shown="True" w212 {
          frame False {
          }
          frame True {
            w231 = "%12.10f" ("format string")
            w252 = TRUE ("append to file? (new file:F)")
            # "Write a summary of the experimental parameters and dichroism to a CSV file."
            # "CSV headers. Commas are needed to keep spacing consistent with row labels and \nthe total number of columns."
            # "Convert matrix of doubles into a matrix of properly formatted strings. This is necessary to \nprepend the row labels, which are strings."
            # "Row labels."
            # "Export data associated with experiment not covered during the data \ncollection process."
            n112 = local read "Reference Averages"() -> (w331:T2)
            n113 = local read "Sample Averages"() -> (w329:T2)
            n114 = local read "Sample Analysis"() -> (w327:T4)
            n115 = local read "Reference Analysis"() -> (w335:T5)
            n116 = Unbundle By Name(w331) -> ("Channel 1"=w330:T11, "Channel 2"=w316:T11, "Channel 3"=w312:T11)
            n117 = Unbundle By Name(w329) -> ("Channel 1"=w300:T11, "Channel 2"=w291:T11, "Channel 3"=w290:T11)
            n118 = Unbundle By Name(w327) -> ("Channel 1"=w328:T12, "Channel 2"=w285:T12, "Channel 3"=w282:T12)
            n119 = Unbundle By Name(w335) -> ("Channel 1"=w334:cluster{"I_par":dbl, "I_perp":dbl}, "Channel 2"=w333:cluster{"I_par":dbl, "I_perp":dbl}, "Channel 3"=w332:cluster{"I_par":dbl, "I_perp":dbl})
            n120 = Unbundle By Name(w282) -> ("I_par"=w284:dbl, "I_perp"=w283:dbl, "Dichroic Ratio"=w232:dbl, "Angle (Degrees)"=w213:dbl)
            n121 = Unbundle By Name(w312) -> ("PMT Voltage (V)"=w302:dbl, "Photodiode Voltage (V)"=w315:dbl, "RMS Voltage (V)"=w314:dbl, "Theta (Degrees)"=w313:dbl)
            n122 = Unbundle By Name(w300) -> ("PMT Voltage (V)"=w301:dbl, "Photodiode Voltage (V)"=w303:dbl, "RMS Voltage (V)"=w304:dbl, "Theta (Degrees)"=w305:dbl)
            n123 = Unbundle By Name(w291) -> ("PMT Voltage (V)"=w299:dbl, "Photodiode Voltage (V)"=w298:dbl, "RMS Voltage (V)"=w297:dbl, "Theta (Degrees)"=w296:dbl)
            n124 = Unbundle By Name(w290) -> ("PMT Voltage (V)"=w292:dbl, "Photodiode Voltage (V)"=w293:dbl, "RMS Voltage (V)"=w294:dbl, "Theta (Degrees)"=w295:dbl)
            n125 = Unbundle By Name(w328) -> ("I_par"=w289:dbl, "I_perp"=w288:dbl, "Dichroic Ratio"=w245:dbl, "Angle (Degrees)"=w215:dbl)
            n126 = Unbundle By Name(w285) -> ("I_par"=w286:dbl, "I_perp"=w287:dbl, "Dichroic Ratio"=w233:dbl, "Angle (Degrees)"=w214:dbl)
            n127 = Unbundle By Name(w330) -> ("PMT Voltage (V)"=w324:dbl, "Photodiode Voltage (V)"=w323:dbl, "RMS Voltage (V)"=w322:dbl, "Theta (Degrees)"=w321:dbl)
            n128 = Unbundle By Name(w316) -> ("PMT Voltage (V)"=w317:dbl, "Photodiode Voltage (V)"=w318:dbl, "RMS Voltage (V)"=w319:dbl, "Theta (Degrees)"=w320:dbl)
            n129 = Unbundle By Name(w334) -> ("I_par"=w311:dbl, "I_perp"=w310:dbl)
            n130 = Unbundle By Name(w333) -> ("I_par"=w309:dbl, "I_perp"=w308:dbl)
            n131 = Unbundle By Name(w332) -> ("I_par"=w307:dbl, "I_perp"=w306:dbl)
            n132 = Build Array(w311, w310) -> (w280:dbl[])
            n133 = Build Array(w309, w308) -> (w278:dbl[])
            n134 = Build Array(w307, w306) -> (w276:dbl[])
            n135 = Build Array(w284, w283, w232, w213) -> (w270:dbl[])
            n136 = Build Array(w286, w287, w233, w214) -> (w272:dbl[])
            n137 = Build Array(w289, w288, w245, w215) -> (w274:dbl[])
            n138 = Build Array(w324, w323, w322, w321) -> (w281:dbl[])
            n139 = Build Array(w302, w315, w314, w313) -> (w277:dbl[])
            n140 = Build Array(w301, w303, w304, w305) -> (w275:dbl[])
            n141 = Build Array(w299, w298, w297, w296) -> (w273:dbl[])
            n142 = Build Array(w292, w293, w294, w295) -> (w271:dbl[])
            n143 = Build Array(w317, w318, w319, w320) -> (w279:dbl[])
            n144 = Insert Into Array(array=w281, new element=w280) -> (w269:dbl[])  [unwired: 1 in]
            n145 = Insert Into Array(array=w279, new element=w278) -> (w268:dbl[])  [unwired: 1 in]
            n146 = Insert Into Array(array=w277, new element=w276) -> (w267:dbl[])  [unwired: 1 in]
            n147 = Insert Into Array(array=w275, new element=w274) -> (w266:dbl[])  [unwired: 1 in]
            n148 = Insert Into Array(array=w273, new element=w272) -> (w265:dbl[])  [unwired: 1 in]
            n149 = Insert Into Array(array=w271, new element=w270) -> (w264:dbl[])  [unwired: 1 in]
            n150 = Build Array(w269, w268, w267, w266, w265, w264) -> (w257:T13)
            n151 = Transpose Matrix(1:w257) -> (0:w251:T13)
            n152 = for {
              tunnel: w251 -> [w354] mode=indexing
              tunnel: [w353] -> _ mode=indexing
              shift-right: [w349] -> w254
              shift-left: string[][] [] -> [w351]
              n153 = for {
                tunnel: w354 -> [w359] mode=indexing
                tunnel: [w359] -> w353 mode=indexing
                shift-right: [w355] -> w350
                shift-left: string[] [] -> [w357]
                n154 = Format Into String(format string="%12.10f", w359) -> (resulting string=w356:string)  [unwired: 2 in, 1 out]
                n155 = Build Array (concatenate)(w357, w356) -> (w355:string[])
              }
              n156 = Build Array (concatenate)(w351, w350) -> (w349:string[][])
            }
            n157 = Get Date/Time In Seconds() -> (seconds since 1Jan1904=w242:timestamp)
            n158 = Initialize Array("", -1 ("dimension size"), -1 ("dimension size")) -> (w235:string[][])
            n159 = Get Date/Time String(seconds (now)=w242) -> (date string=w241:string, time string=w240:string)  [unwired: 2 in]
            n160 = Concatenate Strings(w241, w240) -> (w238:string)
            n161 = Build Array("Date", w238) -> (w234:string[])
            n162 = Build Array (concatenate)(w235, w234) -> (w223:string[][])
            n163 = Format Into String(format string=w231, w214) -> (resulting string=w216:string)  [unwired: 2 in, 1 out]
            n164 = Format Into String(format string=w231, w215) -> (resulting string=w228:string)  [unwired: 2 in, 1 out]
            n165 = Format Into String(format string=w231, w213) -> (resulting string=w230:string)  [unwired: 2 in, 1 out]
            n166 = control-ref of="Experimental Parameters"() -> (w244:refnum<vi>)
            n167 = Build Array("Orientation angle (channel 1):", w228) -> (w226:string[])
            n168 = Build Array("Orientation angle (channel 2):", w216) -> (w225:string[])
            n169 = Build Array("Orientation angle (channel 3):", w230) -> (w224:string[])
            n170 = property class="Clust (strict)"(reference=w244) -> ("Controls[]"=w243:refnum<vi>[])  [unwired: 1 in, 2 out]
            n171 = local read "Output Filename (stem)"() -> (w338:path)
            n172 = Build Array (concatenate)(string[] ["Avg. PMT Voltage (V)", "Avg. Photodiode Voltage (V)", "Avg. RMS Voltage (V)", "Avg. Theta (Degrees)", "I parallel", "I perpendicular", "Dichroic Ratio", "Orientation Angle (Degrees)"], w254) -> (w253:string[][])
            n173 = Path To String(path=w338) -> (string=w337:string)
            n174 = Concatenate Strings(w337, "_analysis.csv") -> (w326:string)
            n175 = for {
              tunnel: w243 -> [w348] mode=indexing
              tunnel: [w348] -> _ mode=indexing
              shift-right: [w342] -> w222
              shift-left: w223 -> [w346]
              n176 = property class="Ctl"(reference=w348) -> ("Label.Text"=w345:string, "Value"=w341:variant)  [unwired: 1 in, 2 out]
              n177 = Variant To Data(type=0.0, Variant=w341) -> (data=w339:dbl)  [unwired: 1 in, 1 out]
              n178 = Format Into String(format string="%12.10f", w339) -> (resulting string=w344:string)  [unwired: 2 in, 1 out]
              n179 = Build Array(w345, w344) -> (w343:string[])
              n180 = Build Array (concatenate)(w346, w343) -> (w342:string[][])
            }
            n181 = String To Path(string=w326) -> (path=w325:path)
            n182 = Build Array(",Reference,,,Sample,,,", ",Channel 1,Channel 2,Channel 3,Channel 1,Channel 2, Channel 3") -> (w259:string[])
            n183 = call-poly <vilib>:"Write Delimited Spreadsheet.vi"("file path (dialog if empty)"=w325, "1D data"=w259, "delimiter (\\t)"="\n" ("delimiter (\\t)")) -> ("new file path (Not A Path if cancelled)"=w263:path)  [unwired: 11 in, 1 out]
            n184 = call-poly <vilib>:"Write Delimited Spreadsheet.vi"("file path (dialog if empty)"=w263, "2D data"=w253, "append to file? (new file:F)"=w252, "transpose? (no:F)"=w252, "delimiter (\\t)"="," ("delimiter (\\t)")) -> ()  [unwired: 9 in, 2 out]
            n185 = local read "Output Filename (stem)"() -> (w247:path)
            n186 = Path To String(path=w247) -> (string=w248:string)
            n187 = Concatenate Strings(w248, "_summary.csv") -> (w250:string)
            n188 = String To Path(string=w250) -> (path=w246:path)
            n189 = Build Array (concatenate)(w222, w226, w225, w224) -> (w221:string[][])
            n190 = call-poly <vilib>:"Write Delimited Spreadsheet.vi"("file path (dialog if empty)"=w246, "2D data"=w221, "transpose? (no:F)"=FALSE, "delimiter (\\t)"="," ("delimiter (\\t)")) -> ()  [unwired: 10 in, 2 out]
          }
        }
      }
      event Timeout {
        # "If we are currently collecting \ndata, the user should not be \nable to change controls."
        n191 = event-data() -> ()  [unwired: 1 in, 3 out]
        n192 = local read "Running"() -> (w366:bool)
        n193 = case shown="False" w366 {
          tunnel: w365 -> [w374 _]
          tunnel: w364 -> [w373 _]
          tunnel: w363 -> [w372 _]
          tunnel: w362 -> [w371 _]
          tunnel: w361 -> [w370 _]
          tunnel: w360 -> [w369 _]
          frame False {
            w376 = T7."Disabled and Grayed Out" ("Disabled")
            w377 = T7."Enabled" ("Disabled")
            # "Allow user to adjust the position of the translation stage and manipulate the shutter."
            # "In \"Reference\" mode, the program should store \ndata in the reference indicators. In the \"Sample\" \nmode, the sample indicators should be used. \nThis allows the calculation of the dichroic ratio, \nand hence the dipole orientation."
            n194 = event shown="[1] Timeout" {
              selector: _ -> [_ _]
              dyn-events: _ -> [_ _]
              timeout: 100 -> [_ _]
              tunnel: [w555 _] -> _
              tunnel: w370 -> [w555 _]
              tunnel: w369 -> [w554 _]
              tunnel: [w549 _] -> _
              tunnel: [w548 _] -> _
              event "Shutter Control": Value Change {
                n195 = event-data() -> ("NewVal"=w553:bool)  [unwired: 1 in, 5 out]
                n196 = Select(t=5.0, s=w553, f=0.0) -> (s? t:f=w550:dbl)
                n197 = call "LJUD_eDAC.vi"("Handle In"=w555, "Channel"=0, "Voltage"=w550, "error in"=w554) -> ("Handle Out"=w549:i32, "error out"=w548:errorcluster)  [unwired: 10 in]
              }
              event Timeout {
                n198 = event-data() -> ()  [unwired: 1 in, 3 out]
              }
            }
            n199 = local read "Save Measurements?"() -> (w378:bool)
            n200 = Equal?(x="Data Collection Mode", y=enum32{"Reference", "Sample"}."Sample") -> (x = y?=w383:bool)
            n201 = Select(t=w376, s=w383, f=w377) -> (s? t:f=w381:T7)
            n202 = Select(t=w377, s=w383, f=w376) -> (s? t:f=w380:T7)
            n203 = Select(t=w377, s=w378, f=w376) -> (s? t:f=w379:T7)
            n204 = property on="Output Filename (stem)" class="Path"("DisabledEnum"=w379) -> ()  [unwired: 2 in, 2 out]
            n205 = property on="Selected Reference Channel" class="RadioBtnsControl (strict)"("DisabledEnum"=w381) -> ()  [unwired: 2 in, 2 out]
            n206 = property on="Selected Sample Channel" class="RadioBtnsControl (strict)"("DisabledEnum"=w380) -> ()  [unwired: 2 in, 2 out]
            n207 = while {
              shift-right: [w392] -> _
              shift-left: MCTypedef."idle" -> [w393]
              tunnel: w374 -> [w390]
              tunnel: w373 -> [w389]
              tunnel: w372 -> [w388]
              tunnel: w371 -> [w387]
              tunnel: "Enable Translation Stage" -> [w386]
              stop <- w385 stop-if-true
              n208 = Not(x=w386) -> (.not. x?=w385:bool)
              n209 = case shown="\"forward\"" w393 {
                tunnel: [w394 MCTypedef."idle" MCTypedef."idle" MCTypedef."idle"] -> w392
                tunnel: [_ w444 w477 w513] -> w391
                tunnel: w389 -> [_ w443 w476 w512]
                tunnel: w390 -> [_ w442 w475 w511]
                tunnel: w387 -> [w401 _ _ _]
                tunnel: w388 -> [w399 _ _ _]
                tunnel: [w400 _ _ _] -> _
                frame "idle", Default {
                  n210 = flat-sequence {
                    tunnel: w401 -> [w417]
                    tunnel: w399 -> [w412]
                    tunnel: [w416] -> w398
                    tunnel: [MCTypedef."clear" ("t")] -> w397
                    tunnel: ["clear"] -> w396
                    tunnel: [w403] -> w395
                    tunnel: [w436] -> w400
                    tunnel: w398 -> [w436]
                    tunnel: w397 -> [w434]
                    tunnel: w396 -> [w435]
                    tunnel: w395 -> [w433]
                    tunnel: [w432] -> w394
                    frame #0 {
                      w409 = T14 [enum."DOWN"] items=["0", "1", "2", "3", "4", "5", "6", "7", "8", "9", "A", "B", "C", "D", "E", "F", "G", "H", "I", "J", "K", "L", "M", "N", "O", "P", "Q", "R", "S", "T", "U", "V", "W", "X", "Y", "Z", "F1", "F2", "F3", "F4", "F5", "F6", "F7", "F8", "F9", "F10", "F11", "F12", "F13", "F14", "F15", "ADD", "BACK", "BACKSLASH", "CAPITAL", "COMMA", "DECIMAL", "DELETE", "DIVIDE", "DOWN", "END", "EQUALS", "ESCAPE", "GRAVE (`)", "HOME", "INSERT", "LBRACKET", "LCONTROL", "LEFT", "L ALT", "LSHIFT", "LWIN", "MINUS", "MULTIPLY", "NEXT", "NUMLOCK", "NUMPAD_0", "NUMPAD_1", "NUMPAD_2", "NUMPAD_3", "NUMPAD_4", "NUMPAD_5", "NUMPAD_6", "NUMPAD_7", "NUMPAD_8", "NUMPAD_9", "PAUSE", "PERIOD", "PRIOR (PG UP)", "RBRACKET", "RCONTROL", "RETURN", "RIGHT", "R ALT", "RSHIFT", "RWIN", "SCROLL", "SEMICOLON", "SLASH", "SPACE", "SUBTRACT", "TAB", "UP", "ENTER (num pad)", "' (quote)"] ("y")
                      w415 = T14 [enum."UP"] items=["0", "1", "2", "3", "4", "5", "6", "7", "8", "9", "A", "B", "C", "D", "E", "F", "G", "H", "I", "J", "K", "L", "M", "N", "O", "P", "Q", "R", "S", "T", "U", "V", "W", "X", "Y", "Z", "F1", "F2", "F3", "F4", "F5", "F6", "F7", "F8", "F9", "F10", "F11", "F12", "F13", "F14", "F15", "ADD", "BACK", "BACKSLASH", "CAPITAL", "COMMA", "DECIMAL", "DELETE", "DIVIDE", "DOWN", "END", "EQUALS", "ESCAPE", "GRAVE (`)", "HOME", "INSERT", "LBRACKET", "LCONTROL", "LEFT", "L ALT", "LSHIFT", "LWIN", "MINUS", "MULTIPLY", "NEXT", "NUMLOCK", "NUMPAD_0", "NUMPAD_1", "NUMPAD_2", "NUMPAD_3", "NUMPAD_4", "NUMPAD_5", "NUMPAD_6", "NUMPAD_7", "NUMPAD_8", "NUMPAD_9", "PAUSE", "PERIOD", "PRIOR (PG UP)", "RBRACKET", "RCONTROL", "RETURN", "RIGHT", "R ALT", "RSHIFT", "RWIN", "SCROLL", "SEMICOLON", "SLASH", "SPACE", "SUBTRACT", "TAB", "UP", "ENTER (num pad)", "' (quote)"] ("y")
                      n211 = call-poly <vilib>:"Acquire Input Data.vi"("device ID"=w417, "error in (no error)"=w412) -> ("device ID"=w416:refnum<k1>, "keys pressed"=w408:T14)  [unwired: 15 in, 1 out]
                      n212 = Equal?(x=w408, y=w415) -> (x = y?=w414:bool[])
                      n213 = Index Array(array=w414, index=0) -> (element=w407:bool)
                      n214 = Equal?(x=w408, y=w409) -> (x = y?=w410:bool[])
                      n215 = Index Array(array=w410, index=0) -> (element=w406:bool)
                      n216 = Select(t=1, s=w407, f=0) -> (s? t:f=w426:i32)
                      n217 = Select(t=2, s=w406, f=0) -> (s? t:f=w425:i32)
                      n218 = Or(x=w426, y=w425) -> (x .or. y?=w424:i32)
                      n219 = Equal?(x=w424, y=1) -> (x = y?=w422:bool)
                      n220 = Select(t=MCTypedef."forward", s=w422, f=MCTypedef."reverse") -> (s? t:f=w418:T8)
                      n221 = Exclusive Or(1:w406, 2:w407) -> (0:w431:bool)
                      n222 = Select(t=w418, s=w431, f=MCTypedef."idle") -> (s? t:f=w403:T8)
                    }
                    frame #1 {
                      n223 = Select(t=w434, s=w435, f=w433) -> (s? t:f=w432:T8)
                    }
                  }
                  n224 = Wait (ms)(milliseconds to wait=u32 50) -> ()  [unwired: 1 out]
                }
                frame "forward" {
                  n225 = Multiply(x="sp33d", y=0.1) -> (x*y=w439:dbl)
                  n226 = Format Into String(format string="%1.2f", w439) -> (resulting string=w437:string)  [unwired: 2 in, 1 out]
                  n227 = flat-sequence {
                    tunnel: [w459] -> w449
                    tunnel: [w458] -> w448
                    tunnel: w443 -> [w452]
                    tunnel: w442 -> [w451]
                    tunnel: w437 -> [w450]
                    tunnel: w449 -> [w465]
                    tunnel: w448 -> [w464]
                    tunnel: [w463] -> w447
                    tunnel: [w462] -> w446
                    tunnel: w447 -> [w468]
                    tunnel: w446 -> [w469]
                    tunnel: [w467] -> _
                    tunnel: [w466] -> w444
                    frame #0 {
                      (unwired) "1.0" ("string")
                      n228 = call <vilib>:"Space Constant.vi"() -> ("String"=w453:string)
                      n229 = Concatenate Strings("jog2" ("string"), w453, w450, "\r", "\n") -> (w454:string)
                      n230 = VISA Write(VISA resource name=w452, write buffer=w454, error in (no error)=w451) -> (VISA resource name out=w459:refnum<visa-resource-name>, error out=w458:errorcluster)  [unwired: 1 out]
                    }
                    frame #1 {
                      n231 = VISA Read(VISA resource name=w465, byte count=u32 1024, error in (no error)=w464) -> (VISA resource name out=w463:refnum<visa-resource-name>, read buffer=→"read buffer":string, error out=w462:errorcluster)  [unwired: 1 out]
                    }
                    frame #2 {
                      n232 = VISA Flush I/O Buffer(VISA resource name=w468, error in (no error)=w469) -> (VISA resource name out=w467:refnum<visa-resource-name>, error out=w466:errorcluster)  [unwired: 1 in]
                    }
                  }
                }
                frame "reverse" {
                  n233 = local read "sp33d"() -> (w471:dbl)
                  n234 = Multiply(x=w471, y=-0.1) -> (x*y=w474:dbl)
                  n235 = Format Into String(format string="%1.2f", w474) -> (resulting string=w470:string)  [unwired: 2 in, 1 out]
                  n236 = flat-sequence {
                    tunnel: [w492] -> w482
                    tunnel: [w491] -> w481
                    tunnel: w476 -> [w485]
                    tunnel: w475 -> [w484]
                    tunnel: w470 -> [w483]
                    tunnel: w482 -> [w498]
                    tunnel: w481 -> [w497]
                    tunnel: [w496] -> w480
                    tunnel: [w495] -> w479
                    tunnel: w480 -> [w501]
                    tunnel: w479 -> [w502]
                    tunnel: [w500] -> _
                    tunnel: [w499] -> w477
                    frame #0 {
                      n237 = call <vilib>:"Space Constant.vi"() -> ("String"=w486:string)
                      n238 = Concatenate Strings("jog2" ("string"), w486, w483, "\r", "\n") -> (w487:string)
                      n239 = VISA Write(VISA resource name=w485, write buffer=w487, error in (no error)=w484) -> (VISA resource name out=w492:refnum<visa-resource-name>, error out=w491:errorcluster)  [unwired: 1 out]
                    }
                    frame #1 {
                      n240 = VISA Read(VISA resource name=w498, byte count=u32 1024, error in (no error)=w497) -> (VISA resource name out=w496:refnum<visa-resource-name>, read buffer=w493:string, error out=w495:errorcluster)  [unwired: 1 out]
                      n241 = local write "read buffer"(w493) -> ()
                    }
                    frame #2 {
                      n242 = VISA Flush I/O Buffer(VISA resource name=w501, error in (no error)=w502) -> (VISA resource name out=w500:refnum<visa-resource-name>, error out=w499:errorcluster)  [unwired: 1 in]
                    }
                  }
                }
                frame "clear" {
                  n243 = flat-sequence {
                    tunnel: [w523] -> w506
                    tunnel: [w522] -> w504
                    tunnel: w512 -> [w518]
                    tunnel: w511 -> [w517]
                    tunnel: w506 -> [w527]
                    tunnel: [w525] -> w505
                    tunnel: w504 -> [w526]
                    tunnel: [w524] -> w503
                    tunnel: w505 -> [w533]
                    tunnel: w503 -> [w532]
                    tunnel: [w531] -> w509
                    tunnel: [w528] -> w507
                    tunnel: [w542] -> w510
                    tunnel: w509 -> [w541]
                    tunnel: [w540] -> w508
                    tunnel: w507 -> [w534]
                    tunnel: w510 -> [w545]
                    tunnel: w508 -> [w546]
                    tunnel: [w544] -> _
                    tunnel: [w543] -> w513
                    frame #0 {
                      n244 = call <vilib>:"Space Constant.vi"() -> ("String"=w519:string)
                      n245 = Concatenate Strings("stop2" ("string"), w519, "\r", "\n") -> (w520:string)
                      n246 = VISA Write(VISA resource name=w518, write buffer=w520, error in (no error)=w517) -> (VISA resource name out=w523:refnum<visa-resource-name>, error out=w522:errorcluster)  [unwired: 1 out]
                    }
                    frame #1 {
                      n247 = VISA Flush I/O Buffer(VISA resource name=w527, error in (no error)=w526) -> (VISA resource name out=w525:refnum<visa-resource-name>, error out=w524:errorcluster)  [unwired: 1 in]
                    }
                    frame #2 {
                      n248 = VISA Read(VISA resource name=w533, byte count=u32 1024, error in (no error)=w532) -> (VISA resource name out=w528:refnum<visa-resource-name>, read buffer=w529:string, error out=w531:errorcluster)  [unwired: 1 out]
                      n249 = local write "read buffer"(w529) -> ()
                    }
                    frame #3 {
                      n250 = call <vilib>:"Space Constant.vi"() -> ("String"=w537:string)
                      n251 = Concatenate Strings("*cls" ("string"), w537, "\r", "\n") -> (w535:string)
                      n252 = VISA Write(VISA resource name=w534, write buffer=w535, error in (no error)=w541) -> (VISA resource name out=w542:refnum<visa-resource-name>, error out=w540:errorcluster)  [unwired: 1 out]
                    }
                    frame #4 {
                      n253 = VISA Flush I/O Buffer(VISA resource name=w545, error in (no error)=w546) -> (VISA resource name out=w544:refnum<visa-resource-name>, error out=w543:errorcluster)  [unwired: 1 in]
                    }
                  }
                }
              }
              "error out" <- w391
            }
          }
          frame True {
          }
        }
      }
    }
  }
